vi "check license.vi"(11 "created path":path=path "C:/Data Laser Grade/config") -> ()   [LabVIEW 2024]
uses:
  <vilib>/Utility/error.llb/DialogType.ctl
  rpcrt4.dll
panel:
  out "This PC mac":string
  out "NOt valid":bool
  out "data":timestamp
  out "text":string
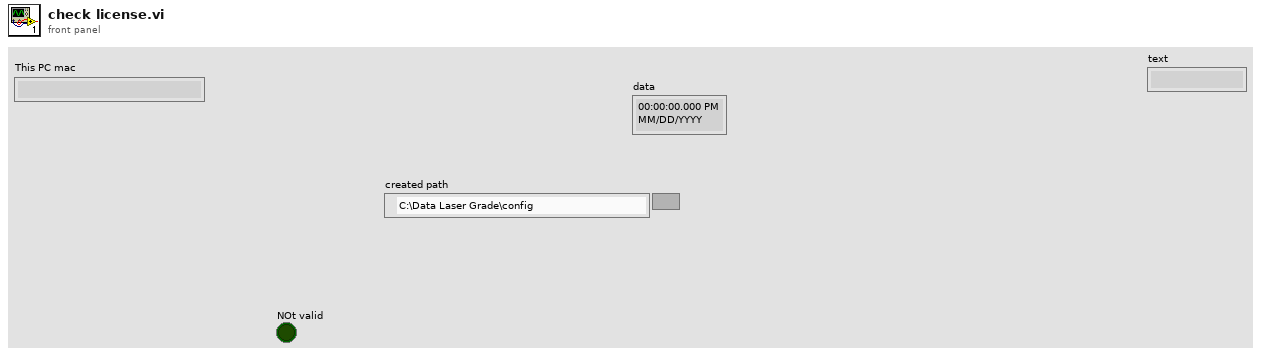
[diagram p1: front panel]
types:
  T1 = enum16{"open", "replace", "create", "open or create", "replace or create", "replace or create with confirmation"}
  T2 = typedef "DialogType.ctl" = u16
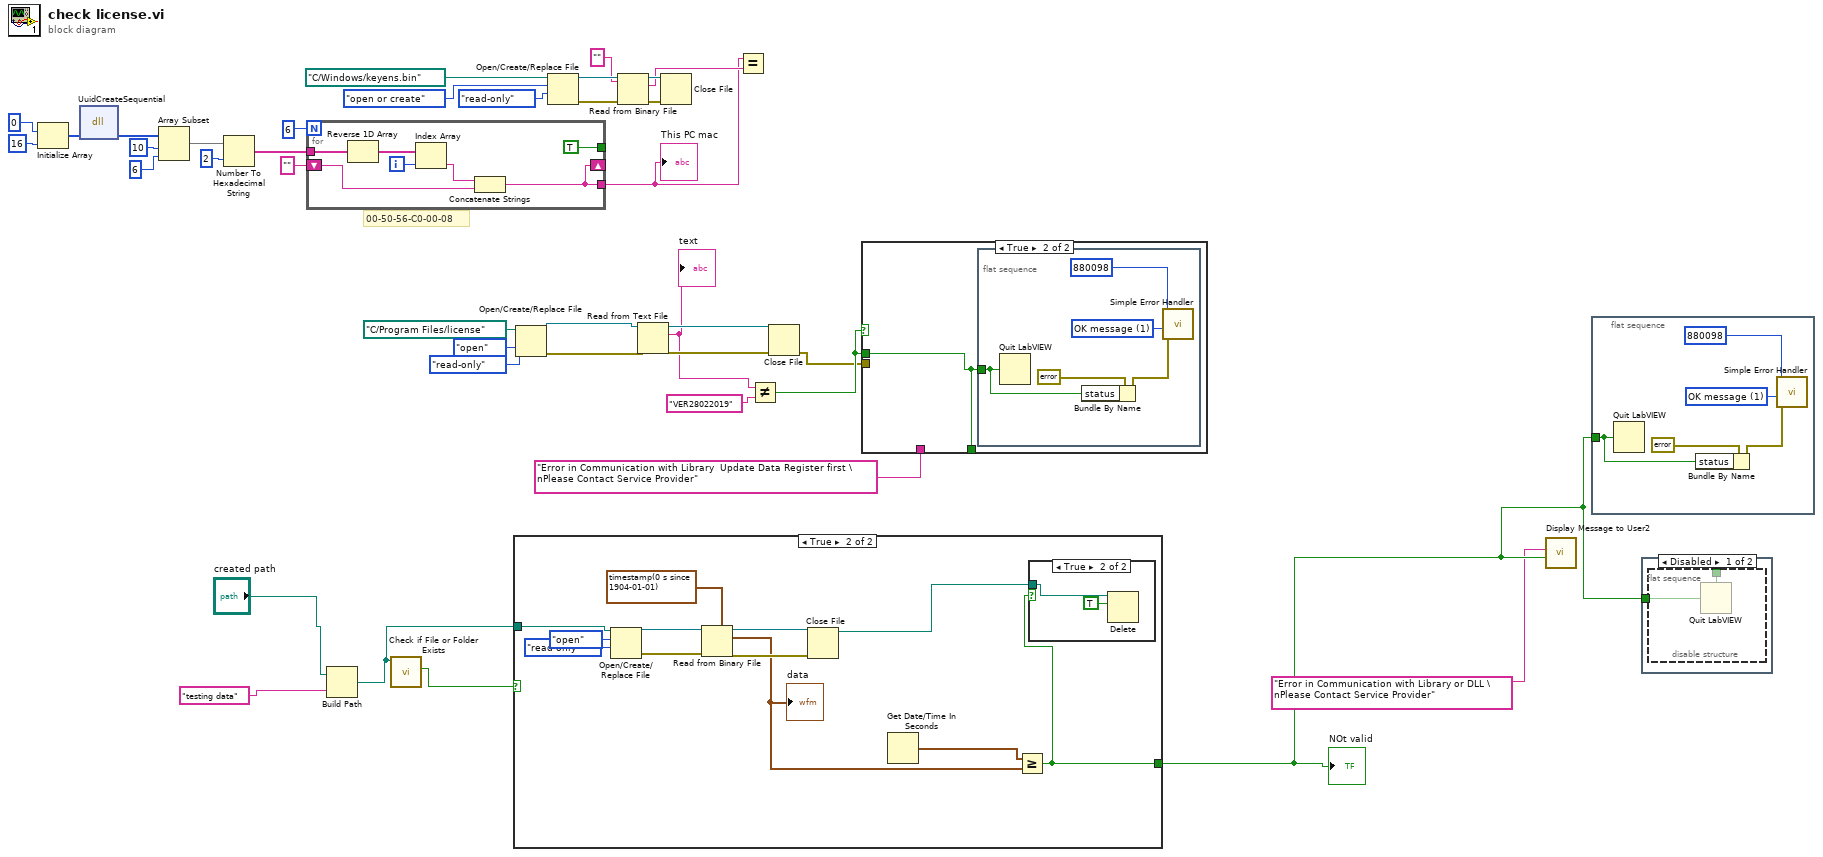
[diagram p0: block diagram]
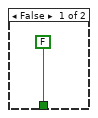
[diagram p3: hidden frame]
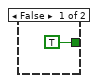
[diagram p4: hidden frame]
diagram:
  # "00-50-56-C0-00-08"
  n1 = Initialize Array(u8 0 ("uuid"), 16 ("dimension size")) -> (w20:u8[])
  n2 = dll-call lib="rpcrt4.dll" fn="UuidCreateSequential"("uuid"=w20) -> ("uuid"=w19:u8[])  [unwired: 4 in, 2 out]
  n3 = Array Subset(array=w19, index=10, length=6) -> (w18:u8[])
  n4 = Number To Hexadecimal String(1:i16 2 ("width (-)"), 2:w18) -> (0:w16:string[])
  n5 = for {
    N: 6 -> [_]
    tunnel: w16 -> [w42]
    shift-right: [w43] -> _
    shift-left: "" -> [w44]
    tunnel: [w43] -> w2
    tunnel: [TRUE] -> _
    i -> [w46]
    n6 = Reverse 1D Array(array=w42) -> (reversed array=w41:string[])
    n7 = Index Array(array=w41, index=w46) -> (element=w45:string)
    n8 = Concatenate Strings(w45, w44) -> (w43:string)
  }
  "This PC mac" <- w2
  n9 = Build Path(base path="created path", name or relative path="testing data" ("Test Setting")) -> (appended path=w34:path)
  n10 = call <vilib>:"Check if File or Folder Exists.vi"("path"=w34) -> ("file or folder exists?"=w39:bool)  [unwired: 8 in, 2 out]
  n11 = case shown="True" w39 {
    tunnel: w34 -> [_ w51]
    tunnel: [TRUE w48] -> w38
    frame False {
    }
    frame True {
      n12 = Open/Create/Replace File(file path (use dialog)=w51, operation (0:open)=T1."open", access (0:read/write)=enum16{"read/write", "read-only", "write-only"}."read-only") -> (refnum out=w58:refnum<file>, error out=w55:errorcluster)  [unwired: 3 in, 1 out]
      n13 = Read from Binary File(5:timestamp(0 s since 1904-01-01) ("calbration date"), 8:w55, 11:w58) -> (0:w56:errorcluster, 2:w52:timestamp, 3:w57:refnum<file>)  [unwired: 3 in, 1 out]
      "data" <- w52
      n14 = Close File(refnum=w57, error in=w56) -> (path=w49:path)  [unwired: 1 out]
      n15 = Get Date/Time In Seconds() -> (seconds since 1Jan1904=w59:timestamp)
      n16 = Greater Or Equal?(x=w59, y=w52) -> (x >= y?=w48:bool)
      n17 = case shown="True" w48 {
        tunnel: w49 -> [_ w61]
        frame False {
        }
        frame True {
          n18 = Delete(path (use dialog)=w61, entire hierarchy (F)=TRUE) -> ()  [unwired: 3 in, 3 out]
        }
      }
    }
  }
  "NOt valid" <- w38
  n19 = Open/Create/Replace File(file path (use dialog)=path "C:/Program Files/license", operation (0:open)=T1."open", access (0:read/write)=enum16{"read/write", "read-only", "write-only"}."read-only") -> (refnum out=w33:refnum<file>, error out=w30:errorcluster)  [unwired: 3 in, 1 out]
  n20 = Open/Create/Replace File(file path (use dialog)=path "C:/Windows/keyens.bin", operation (0:open)=T1."open or create", access (0:read/write)=enum16{"read/write", "read-only", "write-only"}."read-only") -> (refnum out=w11:refnum<file>, error out=w10:errorcluster)  [unwired: 3 in, 1 out]
  n21 = Read from Binary File(5:"" ("data type"), 8:w10, 11:w11) -> (0:w9:errorcluster, 2:w3:string, 3:w8:refnum<file>)  [unwired: 3 in, 1 out]
  n22 = Read from Text File(file (use dialog)=w33, error in=w30) -> (refnum out=w32:refnum<file>, text=w25:string, error out=w31:errorcluster)  [unwired: 2 in, 1 out]
  "text" <- w25
  n23 = Close File(refnum=w8, error in=w9) -> ()  [unwired: 2 out]
  n24 = Equal?(x=w2, y=w3) -> ()  [unwired: 1 out]
  n25 = Not Equal?(x=w25, y="VER28022019" ("text 2")) -> (x != y?=w24:bool)
  n26 = Close File(refnum=w32, error in=w31) -> (error out=w23:errorcluster)  [unwired: 1 out]
  n27 = case shown="True" w24 {
    tunnel: "Error in Communication with Library  Update Data Register first \nPlease Contact Service Provider" ("error source (\" \")") -> [_ _]
    tunnel: w24 -> [_ w63]
    tunnel: w23 -> [_ _]
    tunnel: [FALSE ("OK") w63] -> _
    frame False {
    }
    frame True {
      n28 = flat-sequence {
        tunnel: w63 -> [w64]
        frame #0 {
          w65 = T2 1 items=["no dialog", "OK message", "continue or stop message", "OK message + warnings", "continue/stop + warnings"] ("type of dialog (OK msg:1)")
          n29 = Quit LabVIEW(quit? (T)=w64) -> ()
          n30 = Bundle By Name(cluster=errorcluster {"status"=TRUE, "code"=880098, "source"=""} ("error in (no error)"), "status"=w64) -> (w68:errorcluster)
          n31 = call <vilib>:"Simple Error Handler.vi"("error code (no error:0)"=880098, "type of dialog (OK msg:1)"=w65, "error in (no error)"=w68) -> ()  [unwired: 2 in, 5 out]
        }
      }
    }
  }
  n32 = call "Display Message to User2"("Enable"=w38, "Message"="Error in Communication with Library or DLL \nPlease Contact Service Provider" ("error source (\" \")")) -> ()  [unwired: 8 in, 2 out]
  n33 = flat-sequence {
    tunnel: w38 -> [w69]
    frame #0 {
      w70 = T2 1 items=["no dialog", "OK message", "continue or stop message", "OK message + warnings", "continue/stop + warnings"] ("type of dialog (OK msg:1)")
      n34 = Quit LabVIEW(quit? (T)=w69) -> ()
      n35 = Bundle By Name(cluster=errorcluster {"status"=TRUE, "code"=880098, "source"=""} ("error in (no error)"), "status"=w69) -> (w73:errorcluster)
      n36 = call <vilib>:"Simple Error Handler.vi"("error code (no error:0)"=880098, "type of dialog (OK msg:1)"=w70, "error in (no error)"=w73) -> ()  [unwired: 2 in, 5 out]
    }
  }
  n37 = flat-sequence {
    tunnel: w38 -> [w74]
    frame #0 {
      n38 = disable-structure shown="Disabled" {
        disable-tunnel: w74 -> [w75 _]
        frame Disabled {
          n39 = Quit LabVIEW(quit? (T)=w75) -> ()
        }
        frame Enabled {
        }
      }
    }
  }
